vi "SYST_ACT_MEAS.vi"(0 "VISA IN":refnum<visa-resource-name>, 5 "error in":errorcluster) -> (14 "VISA Out":refnum<visa-resource-name>, 16 "Data":string, 19 "error out":errorcluster)   [LabVIEW 2018, in "PNA-X.lvlib"]
doc: "SYSTem:ACTive:MEASurement? \n(Read-only) Returns the name of the active measurement or an error message if there is no active \nmeasurement. While looking at the PNA display, the active measurement is the trace that has an \nindented Trace Status button and a label in the upper-left corner of the display. Only displayed \nmeasurements can be active. \nExamples SYST:PRES \nSYST:ACT:MEAS? \n'Returns \"CH1_S11_1\" \nReturn Type String \nDefault Not Applicable"
uses:
  PNA-X.lvlib
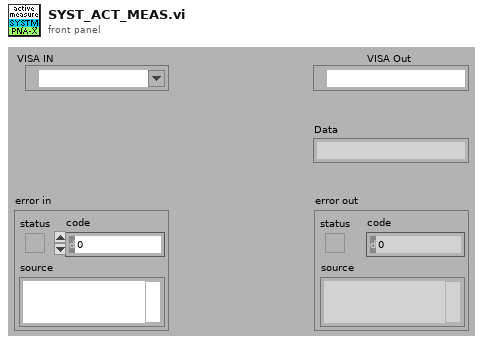
[diagram p1: front panel]
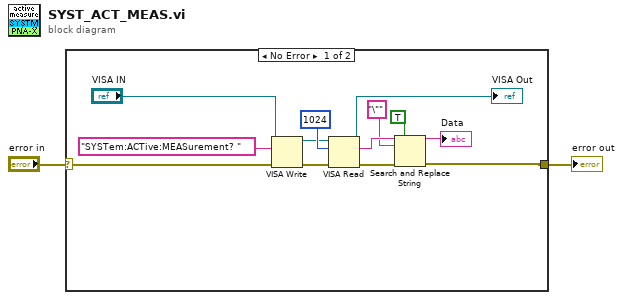
[diagram p0: block diagram]
diagram:
  n1 = case shown="No Error" "error in" {
    selector: "error in" -> [w10 w16]
    tunnel: [w4 w16] -> w1
    frame No Error {
      n2 = VISA Write(VISA resource name="VISA IN", write buffer="SYSTem:ACTive:MEASurement? " ("Cmdline"), error in (no error)=w10) -> (VISA resource name out=w12:refnum<visa-resource-name>, error out=w14:errorcluster)  [unwired: 1 out]
      n3 = VISA Read(VISA resource name=w12, byte count=1024, error in (no error)=w14) -> (VISA resource name out=→"VISA Out":refnum<visa-resource-name>, read buffer=w7:string, error out=w8:errorcluster)  [unwired: 1 out]
      n4 = Search and Replace String(replace all?=TRUE ("replace all? (F)"), input string=w7, search string="\"", error in=w8) -> (result string=→"Data":string, error out=w4:errorcluster)  [unwired: 4 in, 2 out]
    }
    frame Error {
    }
  }
  "error out" <- w1
